vi "GetDiagramImage.vi"(8 "Draw Area Size":T1, 9 "appended path":path, 11 "String":string) -> (3 "2D Picture":picture)   [LabVIEW 2020]
uses:
  <vilib>/Utility/miscctls.llb/LVBoundsTypeDef.ctl
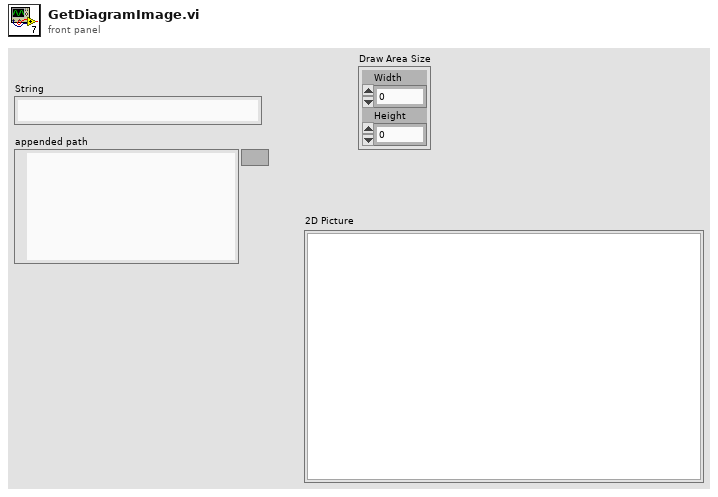
[diagram p1: front panel]
types:
  T1 = typedef "LVBoundsTypeDef.ctl" = cluster{"Width":u32, "Height":u32}
  T2 = typedef "imagedata.ctl" = cluster{"image type":i32, "image depth":i32, "image":u8[], "mask":u8[], "colors":u32[], "Rectangle":cluster{"left":i16, "top":i16, "right":i16, "bottom":i16}}
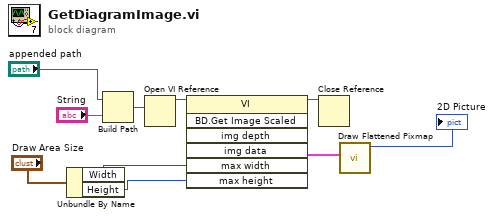
[diagram p0: block diagram]
diagram:
  n1 = Unbundle By Name("Draw Area Size") -> ("Width"=w2:u32, "Height"=w1:u32)
  n2 = Build Path(base path="appended path", name or relative path="String") -> (appended path=w8:path)
  n3 = Open VI Reference(vi path=w8) -> (vi reference=w9:refnum<vi>)  [unwired: 5 in, 1 out]
  n4 = invoke class="VI" method="BD.Get Image Scaled"(reference=w9, "max width"=w2, "max height"=w1) -> (reference out=w10:refnum<vi>, "img data"=w5:T2)  [unwired: 4 in, 5 out]
  n5 = Close Reference(reference=w10) -> ()  [unwired: 1 in, 1 out]
  n6 = call <vilib>:"Draw Flattened Pixmap.vi"("image data"=w5) -> ("new picture"=→"2D Picture":picture)  [unwired: 8 in]
